vi "tirf-release-handle.vi"(11 "handle":i32) -> ()   [LabVIEW 2014]
uses:
  TIRF-Lock_Upgrade/TIRF-Lock/program files/Mad City Labs/TIRF-Lock/TIRF-Lock.dll
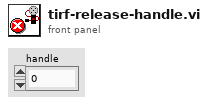
[diagram p1: front panel]
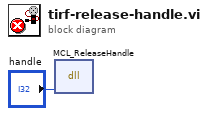
[diagram p0: block diagram]
diagram:
  n1 = dll-call lib="C:/Users/Bakir/Desktop/TIRF-Lock_Upgrade/TIRF-Lock/program files/Mad City Labs/TIRF-Lock/TIRF-Lock.dll" fn="MCL_ReleaseHandle"("handle"="handle") -> ()  [unwired: 4 in, 3 out]
